vi "通讯状态指示.vi"(8 "错误输入（无错误）":errorcluster, 10 "reference":refnum<vi>, 11 "Boolean输入":refnum<vi>) -> ()   [LabVIEW 2016]
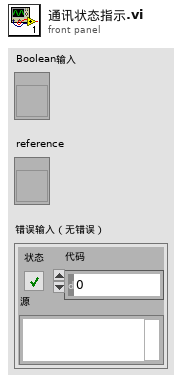
[diagram p1: front panel]
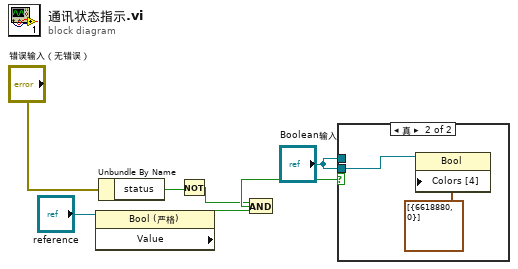
[diagram p0: block diagram]
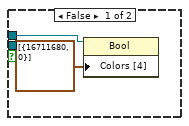
[diagram p2: hidden frame]
diagram:
  n1 = property class="Bool (严格)"(reference="reference") -> ("Value"=w5:bool)  [unwired: 1 in, 2 out]
  n2 = Unbundle By Name("错误输入（无错误）") -> ("status"=w4:bool)
  n3 = Not(x=w4) -> (.not. x?=w6:bool)
  n4 = And(x=w6, y=w5) -> (x .and. y?=w7:bool)
  n5 = case shown="真" w7 {
    tunnel: "Boolean输入" -> [w8 _]
    tunnel: "Boolean输入" -> [_ w10]
    frame False {
      n6 = property on="属性节点" class="Bool"(reference=w8, "Colors [4]"=cluster{u32, u32}[] [{16711680, 0}] ("颜色[4]")) -> ()  [unwired: 1 in, 2 out]
    }
    frame True {
      n7 = property on="属性节点" class="Bool"(reference=w10, "Colors [4]"=cluster{u32, u32}[] [{6618880, 0}] ("颜色[4]")) -> ()  [unwired: 1 in, 2 out]
    }
  }
